vi "weatherdata.vi"() -> ()   [LabVIEW 2018]
panel:
  out "数据":T1(array[cluster])
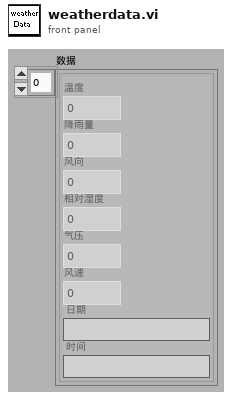
[diagram p1: front panel]
types:
  T1 = cluster{"温度":dbl, "降雨量":dbl, "风向":dbl, "相对湿度":dbl, "气压":dbl, "风速":dbl, "日期":string, "时间":string}[]
diagram:
